vi "Delete_Crossconnection-1.vi"(5 "[IN] Row index\nInitial Point":i32, 7 "[IN] Column in\ndex Initial Point":i32, 9 "[IN] Indicies of Cross\nconnected Points":i32[](array[numeric]), 10 "[IN] The other point \nfor crossconnection found":bool, 11 "[IN] Track group":T1) -> (1 "[OUT] Track group":T1, 2 "[OUT] Column index\nCorrect initial point":i32, 3 "[OUT] Row index\nCorrect initial point":i32)   [LabVIEW 2013]
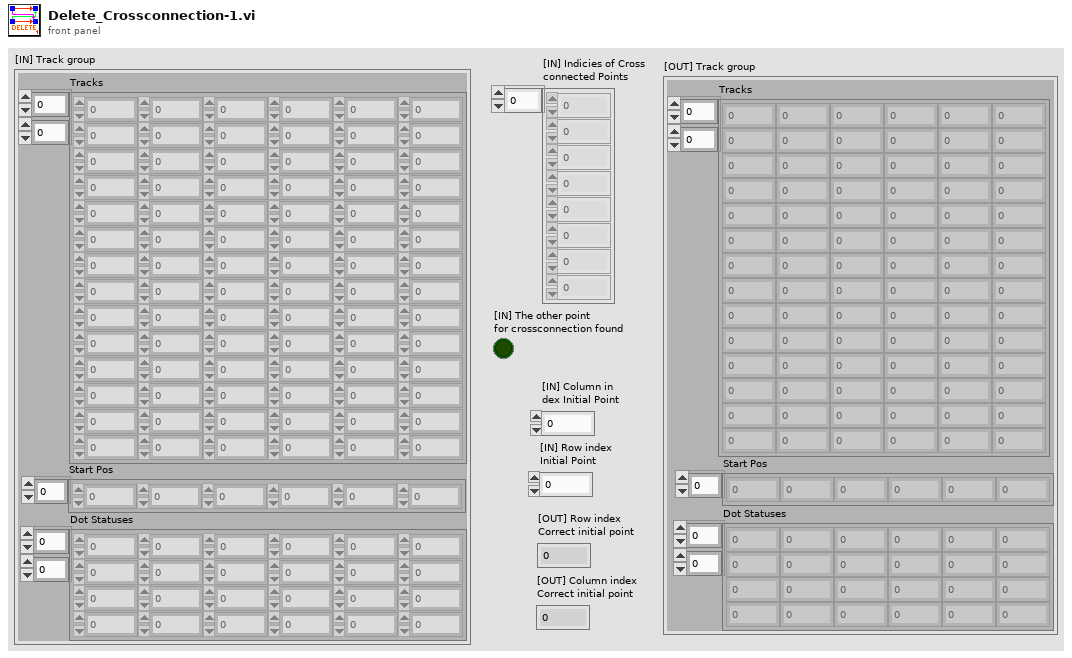
[diagram p1: front panel]
types:
  T1 = cluster{"Tracks":dbl[][], "Start Pos":i32[], "Dot Statuses":i16[][]}
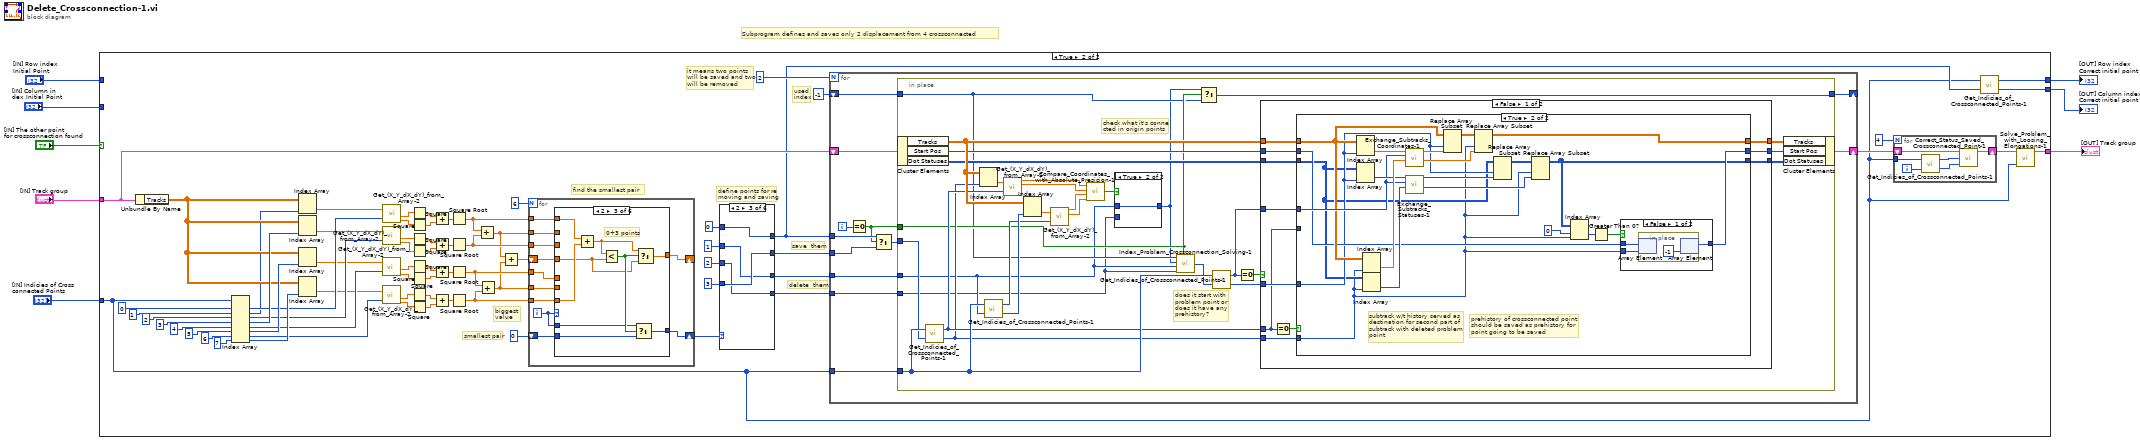
[diagram p0: block diagram]
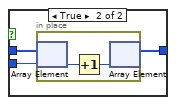
[diagram p4: hidden frame]
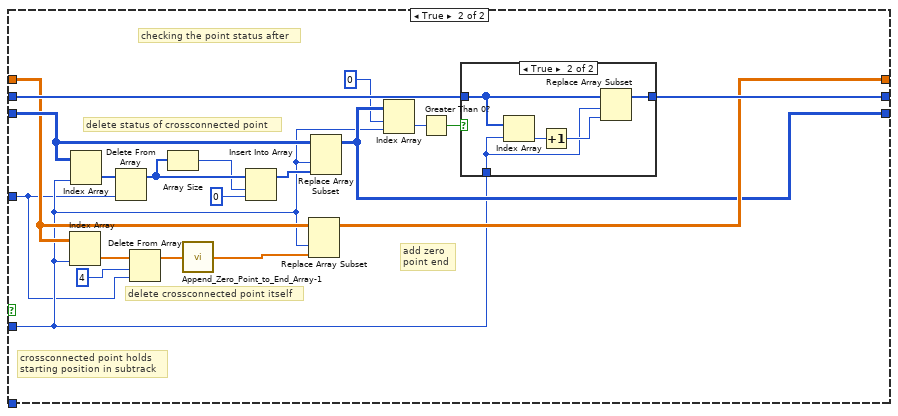
[diagram p5: hidden frame]
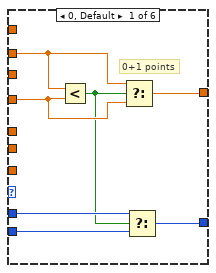
[diagram p13: hidden frame]
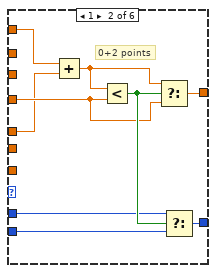
[diagram p14: hidden frame]
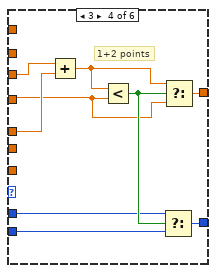
[diagram p15: hidden frame]
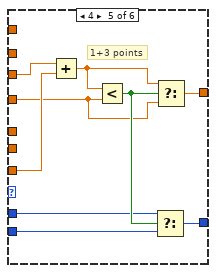
[diagram p16: hidden frame]
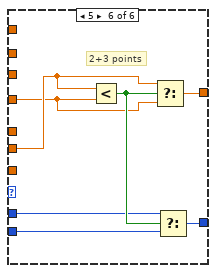
[diagram p17: hidden frame]
diagram:
  # "Subprogram defines and saves only 2 displacement from 4 crossconnected"
  n1 = case shown="True" "[IN] The other point \nfor crossconnection found" {
    tunnel: "[IN] Track group" -> [w11 w25]
    tunnel: "[IN] Indicies of Cross\nconnected Points" -> [_ w14]
    tunnel: [w11 w13] -> w5
    tunnel: [w10 w18] -> w4
    tunnel: [w9 w17] -> w3
    tunnel: "[IN] Row index\nInitial Point" -> [w10 _]
    tunnel: "[IN] Column in\ndex Initial Point" -> [w9 _]
    frame False {
    }
    frame True {
      # "used \nindex"
      # "it means two points\nwill be saved and two\nwill be removed"
      # "define points for re\nmoving and saving"
      # "delete  them"
      # "save  them"
      # "smallest pair"
      # "biggest \nvalue"
      # "find the smallest pair"
      n2 = Unbundle By Name(w25) -> ("Tracks"=w70:dbl[][])
      n3 = Index Array(array=w14, index #1=0 ("index"), index #2=1 ("index"), index #3=2 ("index"), index #4=3 ("index"), index #5=4 ("index"), index #6=5 ("index"), index #7=6 ("index"), index #8=7 ("index")) -> (element #1=w67:i32, element #2=w30:i32, element #3=w65:i32, element #4=w72:i32, element #5=w63:i32, element #6=w71:i32, element #7=w61:i32, element #8=w69:i32)
      n4 = Index Array(array=w70, index (col)=w69) -> (element=w62:dbl[])  [unwired: 1 in]
      n5 = Index Array(array=w70, index (col)=w30) -> (element=w68:dbl[])  [unwired: 1 in]
      n6 = Index Array(array=w70, index (col)=w72) -> (element=w66:dbl[])  [unwired: 1 in]
      n7 = Index Array(array=w70, index (col)=w71) -> (element=w64:dbl[])  [unwired: 1 in]
      n8 = call "Get_(X_Y_dX_dY)_from_Array-2.vi"("(X,Y,dX,dY)"=w66, "Index of Displacement"=w65) -> ("dX"=w52:dbl, "dY"=w51:dbl)  [unwired: 2 out]
      n9 = call "Get_(X_Y_dX_dY)_from_Array-2.vi"("(X,Y,dX,dY)"=w64, "Index of Displacement"=w63) -> ("dX"=w47:dbl, "dY"=w46:dbl)  [unwired: 2 out]
      n10 = call "Get_(X_Y_dX_dY)_from_Array-2.vi"("(X,Y,dX,dY)"=w62, "Index of Displacement"=w61) -> ("dX"=w42:dbl, "dY"=w41:dbl)  [unwired: 2 out]
      n11 = call "Get_(X_Y_dX_dY)_from_Array-2.vi"("(X,Y,dX,dY)"=w68, "Index of Displacement"=w67) -> ("dX"=w57:dbl, "dY"=w56:dbl)  [unwired: 2 out]
      n12 = Square(x=w57) -> (x^2=w60:dbl)
      n13 = Square(x=w56) -> (x^2=w59:dbl)
      n14 = Square(x=w52) -> (x^2=w55:dbl)
      n15 = Square(x=w51) -> (x^2=w54:dbl)
      n16 = Square(x=w47) -> (x^2=w50:dbl)
      n17 = Square(x=w46) -> (x^2=w49:dbl)
      n18 = Square(x=w42) -> (x^2=w45:dbl)
      n19 = Square(x=w41) -> (x^2=w44:dbl)
      n20 = Add(x=w60, y=w59) -> (x+y=w58:dbl)
      n21 = Add(x=w55, y=w54) -> (x+y=w53:dbl)
      n22 = Add(x=w50, y=w49) -> (x+y=w48:dbl)
      n23 = Add(x=w45, y=w44) -> (x+y=w43:dbl)
      n24 = Square Root(x=w58) -> (sqrt(x)=w39:dbl)
      n25 = Square Root(x=w53) -> (sqrt(x)=w38:dbl)
      n26 = Square Root(x=w48) -> (sqrt(x)=w37:dbl)
      n27 = Square Root(x=w43) -> (sqrt(x)=w36:dbl)
      n28 = Add(x=w39, y=w38) -> (x+y=w33:dbl)
      n29 = Add(x=w37, y=w36) -> (x+y=w32:dbl)
      n30 = Add(x=w33, y=w32) -> (x+y=w35:dbl)
      n31 = for {
        N: 6 -> [_]
        tunnel: w39 -> [w233]
        tunnel: w38 -> [w232]
        tunnel: w37 -> [w227]
        tunnel: w36 -> [w226]
        shift-right: [w230] -> _
        shift-left: w35 -> [w235]
        tunnel: w33 -> [w234]
        tunnel: w32 -> [w225]
        shift-right: [w228] -> w31
        shift-left: 0 -> [w229]
        i -> [w231]
        n32 = case shown="2" w231 {
          tunnel: w235 -> [w241 w246 w254 w263 w272 w281]
          tunnel: w234 -> [w242 _ _ _ _ _]
          tunnel: w233 -> [_ w251 w256 _ _ _]
          tunnel: w232 -> [_ _ _ w265 w274 _]
          tunnel: w231 -> [w239 w248 w258 w267 w271 w284]
          tunnel: [w240 w243 w253 w262 w276 w280] -> w230
          tunnel: w229 -> [w238 w247 w257 w266 w270 w283]
          tunnel: [w237 w249 w252 w261 w275 w279] -> w228
          tunnel: w227 -> [_ w244 _ w264 _ _]
          tunnel: w226 -> [_ _ w255 _ w273 _]
          tunnel: w225 -> [_ _ _ _ _ w282]
          frame 0, Default {
            # "0+1 points"
            n33 = Less?(x=w242, y=w241) -> (x < y?=w236:bool)
            n34 = Select(t=w242, s=w236, f=w241) -> (s? t:f=w240:dbl)
            n35 = Select(t=w239, s=w236, f=w238) -> (s? t:f=w237:i32)
          }
          frame 1 {
            # "0+2 points"
            n36 = Add(x=w251, y=w244) -> (x+y=w245:dbl)
            n37 = Less?(x=w245, y=w246) -> (x < y?=w250:bool)
            n38 = Select(t=w245, s=w250, f=w246) -> (s? t:f=w243:dbl)
            n39 = Select(t=w248, s=w250, f=w247) -> (s? t:f=w249:i32)
          }
          frame 2 {
            # "0+3 points"
            n40 = Add(x=w256, y=w255) -> (x+y=w259:dbl)
            n41 = Less?(x=w259, y=w254) -> (x < y?=w260:bool)
            n42 = Select(t=w258, s=w260, f=w257) -> (s? t:f=w252:i32)
            n43 = Select(t=w259, s=w260, f=w254) -> (s? t:f=w253:dbl)
          }
          frame 3 {
            # "1+2 points"
            n44 = Add(x=w265, y=w264) -> (x+y=w268:dbl)
            n45 = Less?(x=w268, y=w263) -> (x < y?=w269:bool)
            n46 = Select(t=w267, s=w269, f=w266) -> (s? t:f=w261:i32)
            n47 = Select(t=w268, s=w269, f=w263) -> (s? t:f=w262:dbl)
          }
          frame 4 {
            # "1+3 points"
            n48 = Add(x=w274, y=w273) -> (x+y=w277:dbl)
            n49 = Less?(x=w277, y=w272) -> (x < y?=w278:bool)
            n50 = Select(t=w271, s=w278, f=w270) -> (s? t:f=w275:i32)
            n51 = Select(t=w277, s=w278, f=w272) -> (s? t:f=w276:dbl)
          }
          frame 5 {
            # "2+3 points"
            n52 = Less?(x=w282, y=w281) -> (x < y?=w285:bool)
            n53 = Select(t=w282, s=w285, f=w281) -> (s? t:f=w280:dbl)
            n54 = Select(t=w284, s=w285, f=w283) -> (s? t:f=w279:i32)
          }
        }
      }
      n55 = case shown="2" w31 {
        tunnel: 0 -> [w204 w208 w212 w214 w218 w222]
        tunnel: 1 -> [w203 w206 w210 w216 w220 w221]
        tunnel: 2 -> [w202 w207 w209 w215 w217 w224]
        tunnel: 3 -> [w201 w205 w211 w213 w219 w223]
        tunnel: [w204 w208 w212 w216 w220 w224] -> w19
        tunnel: [w203 w207 w211 w215 w219 w223] -> w20
        tunnel: [w202 w206 w210 w214 w218 w222] -> w24
        tunnel: [w201 w205 w209 w213 w217 w221] -> w23
        frame 0, Default {
        }
        frame 1 {
        }
        frame 2 {
        }
        frame 3 {
        }
        frame 4 {
        }
        frame 5 {
        }
      }
      n56 = for {
        N: 2 -> [_]
        tunnel: w14 -> [w97]
        tunnel: w19 -> [w92]
        tunnel: w20 -> [w91]
        tunnel: w24 -> [w96]
        tunnel: w23 -> [w95]
        shift-right: [w94] -> w22
        shift-left: w25 -> [w98]
        shift-right: [w88] -> _
        shift-left: -1 -> [w89]
        i -> [w93]
        n57 = Equal To 0?(x=w93) -> (x = 0?=w87:bool)
        n58 = Select(t=w92, s=w87, f=w91) -> (s? t:f=w90:i32)
        n59 = in-place {
          in-place-border: w97 -> [w118]
          in-place-border: w96 -> [w100]
          in-place-border: w95 -> [w99]
          in-place-border: w90 -> [w108]
          in-place-border: w89 -> [w103]
          in-place-border: [w105] -> w88
          in-place-border: w87 -> [w104]
          # "does it start with \nproblem point or\ndoes it have any \nprehistory?"
          # "check what it's conne\ncted in origin points"
          n60 = in-place-cluster #1(w98) -> ("Tracks"=w116:dbl[][], "Start Pos"=w115:i32[], "Dot Statuses"=w114:i16[][])
          n61 = call "Get_Indicies_of_Crossconnected_Points-1.vi"("[IN] Index of point"=w108, "[IN] Indicies of Cross\nconnected Points"=w118) -> ("[OUT] Column index"=w106:i32, "[OUT] Row index"=w107:i32)
          n62 = Index Array(array=w116, index (col)=w106) -> (element=w127:dbl[])  [unwired: 1 in]
          n63 = call "Get_Indicies_of_Crossconnected_Points-1.vi"("[IN] Index of point"=w100, "[IN] Indicies of Cross\nconnected Points"=w118) -> ("[OUT] Column index"=w126:i32, "[OUT] Row index"=w124:i32)
          n64 = call "Get_(X_Y_dX_dY)_from_Array-2.vi"("(X,Y,dX,dY)"=w127, "Index of Displacement"=w107) -> ("X"=w123:dbl, "Y"=w122:dbl)  [unwired: 2 out]
          n65 = Index Array(array=w116, index (col)=w126) -> (element=w125:dbl[])  [unwired: 1 in]
          n66 = call "Get_(X_Y_dX_dY)_from_Array-2.vi"("(X,Y,dX,dY)"=w125, "Index of Displacement"=w124) -> ("X"=w121:dbl, "Y"=w120:dbl)  [unwired: 2 out]
          n67 = call "Compare_Coordinates_with_Absolute_Presicion-1.vi"("X 1"=w123, "Y 1"=w122, "X 2"=w121, "Y 2"=w120) -> ("[OUT] Same coordinates?"=w119:bool)  [unwired: 1 in]
          n68 = case shown="True" w119 {
            tunnel: w100 -> [_ w200]
            tunnel: w99 -> [w199 _]
            tunnel: [w199 w200] -> w102
            frame False {
            }
            frame True {
            }
          }
          n69 = call "Index_Problem_Crossconnection_Solving-1.vi"("[IN] Used Index"=w103, "[IN] Defined Index"=w102, "[IN] 1st Index for Deletion"=w100, "[IN] 2nd Index for Deletion"=w99, "[IN] Is it first step?"=w104) -> ("[OUT] Index of Track wi\nth Point For Deletion"=w101:i32)
          n70 = Select(t=w102, s=w104, f=w103) -> (s? t:f=w105:i32)
          n71 = call "Get_Indicies_of_Crossconnected_Points-1.vi"("[IN] Index of point"=w101, "[IN] Indicies of Cross\nconnected Points"=w118) -> ("[OUT] Column index"=w113:i32, "[OUT] Row index"=w111:i32)
          n72 = Equal To 0?(x=w111) -> (x = 0?=w117:bool)
          n73 = case shown="False" w117 {
            tunnel: w116 -> [w137 w182]
            tunnel: w115 -> [w136 w192]
            tunnel: w114 -> [w135 w187]
            tunnel: w113 -> [w130 w177]
            tunnel: [w133 w191] -> w112
            tunnel: w111 -> [w129 w174]
            tunnel: [w134 w180] -> w110
            tunnel: [w132 w178] -> w109
            tunnel: w107 -> [w128 _]
            tunnel: w106 -> [w131 _]
            frame False {
              n74 = Equal To 0?(x=w128) -> (x = 0?=w138:bool)
              n75 = case shown="True" w138 {
                tunnel: w137 -> [w141 w158]
                tunnel: w136 -> [w140 w149]
                tunnel: w135 -> [w139 w146]
                tunnel: [w141 w154] -> w134
                tunnel: [w140 w147] -> w133
                tunnel: [w139 w145] -> w132
                tunnel: w131 -> [_ w144]
                tunnel: w130 -> [_ w148]
                tunnel: w129 -> [_ w159]
                tunnel: w128 -> [_ _]
                frame False {
                  # "I suppose that tracking algorithm will be able to resolve such problem in this case"
                }
                frame True {
                  # "subtrack w/t history served as \ndestination for second part of \nsubtrack with deleted problem \npoint"
                  # "prehistory of crossconnected point \nshould be saved as prehistory for \npoint going to be saved"
                  n76 = Index Array(array=w158, index (col)=w148) -> (element=w163:dbl[])  [unwired: 1 in]
                  n77 = Index Array(array=w146, index (col)=w148) -> (element=w161:i16[])  [unwired: 1 in]
                  n78 = Index Array(array=w158, index (col)=w144) -> (element=w162:dbl[])  [unwired: 1 in]
                  n79 = Index Array(array=w146, index (col)=w144) -> (element=w160:i16[])  [unwired: 1 in]
                  n80 = call "Exchange_Subtracks_Coordinates-1.vi"("[IN] Subtrack wit\nhout prehistory"=w162, "[IN] Row index \nProblem Point"=w159, "[IN] Subtrack \nwith problem"=w163) -> ("[OUT] Reconnected subtrack\n(posthistory after deleted \ncrossconnected point)"=w155:dbl[], "[OUT] Reconnected subtrack\nPrehistory + alternative prob\nlem point"=w157:dbl[])  [unwired: 3 in]
                  n81 = call "Exchange_Subtracks_Statuses-1.vi"("[IN] Statuses wit\nhout prehistory"=w160, "[IN] Row index \nProblem Point"=w159, "[IN] Statuses\nwith problem"=w161) -> ("[OUT] Reconnected statuses\n(posthistory after deleted \ncrossconnected point)"=w151:i16[], "[OUT] Reconnected statuses\nPrehistory + alternative prob\nlem point"=w153:i16[])  [unwired: 3 in]
                  n82 = Replace Array Subset(array=w158, new element=w157, index (col)=w148) -> (w156:dbl[][])  [unwired: 1 in]
                  n83 = Replace Array Subset(array=w156, new element=w155, index (col)=w144) -> (w154:dbl[][])  [unwired: 1 in]
                  n84 = Replace Array Subset(array=w146, new element=w153, index (col)=w148) -> (w152:i16[][])  [unwired: 1 in]
                  n85 = Replace Array Subset(array=w152, new element=w151, index (col)=w144) -> (w145:i16[][])  [unwired: 1 in]
                  n86 = Index Array(array=w145, index (row)=0 ("disabled index (row)"), index (col)=w144) -> (element=w150:i16)
                  n87 = Greater Than 0?(x=w150) -> (x > 0?=w142:bool)
                  n88 = case shown="False" w142 {
                    tunnel: w149 -> [w166 w170]
                    tunnel: w144 -> [w165 w169]
                    tunnel: [w164 w168] -> w147
                    frame False {
                      n89 = in-place {
                        n90 = in-place-array #2(w166, w165) -> ()  [unwired: 1 out]
                        n91 = in-place-array #2(-1) -> (w164:i32[])  [unwired: 1 out]
                      }
                    }
                    frame True {
                      n92 = in-place {
                        n93 = in-place-array #3(w170, w169) -> (w172:i32)
                        n94 = Increment(x=w172) -> (x+1=w171:i32)
                        n95 = in-place-array #3(w171) -> (w168:i32[])  [unwired: 1 out]
                      }
                    }
                  }
                }
              }
            }
            frame True {
              # "add zero \npoint end"
              # "checking the point status after"
              # "delete crossconnected point itself"
              # "delete status of crossconnected point"
              # "crossconnected point holds \nstarting position in subtrack"
              n96 = Index Array(array=w182, index (col)=w177) -> (element=w185:dbl[])  [unwired: 1 in]
              n97 = Index Array(array=w187, index (col)=w177) -> (element=w190:i16[])  [unwired: 1 in]
              n98 = Delete From Array(array=w190, index=w174) -> (array with subset deleted=w189:i16[])  [unwired: 1 in, 1 out]
              n99 = Delete From Array(array=w185, length=4, index=w174) -> (array with subset deleted=w183:dbl[])  [unwired: 1 out]
              n100 = Array Size(array=w189) -> (size(s)=w179:i32)
              n101 = call "Append_Zero_Point_to_End_Array-1.vi"("[IN] Array with \nDisplacements"=w183) -> ("[OUT] Array with \nAppended Point"=w181:dbl[])
              n102 = Insert Into Array(array=w189, index=w179, new element=i16 0 ("new element/subarray")) -> (w186:i16[])
              n103 = Replace Array Subset(array=w182, new element=w181, index (col)=w177) -> (w180:dbl[][])  [unwired: 1 in]
              n104 = Replace Array Subset(array=w187, new element=w186, index (col)=w177) -> (w178:i16[][])  [unwired: 1 in]
              n105 = Index Array(array=w178, index (row)=0 ("disabled index (row)"), index (col)=w177) -> (element=w176:i16)
              n106 = Greater Than 0?(x=w176) -> (x > 0?=w175:bool)
              n107 = case shown="True" w175 {
                tunnel: w192 -> [w193 w198]
                tunnel: [w193 w195] -> w191
                tunnel: w177 -> [_ w194]
                frame False {
                }
                frame True {
                  n108 = Index Array(array=w198, index=w194) -> (element=w197:i32)
                  n109 = Increment(x=w197) -> (x+1=w196:i32)
                  n110 = Replace Array Subset(array=w198, new element=w196, index=w194) -> (w195:i32[])
                }
              }
            }
          }
          n111 = in-place-cluster #1("Tracks"=w110, "Start Pos"=w112, "Dot Statuses"=w109) -> (w94:T1)
        }
      }
      n112 = for {
        N: 4 -> [_]
        shift-right: [w85] -> w15
        shift-left: w22 -> [w86]
        tunnel: w14 -> [w82]
        i -> [w81]
        n113 = call "Get_Indicies_of_Crossconnected_Points-1.vi"("[IN] Index of point"=w81, "[IN] Indicies of Cross\nconnected Points"=w82) -> ("[OUT] Column index"=w83:i32, "[OUT] Row index"=w84:i32)
        n114 = call "Correct_Status_Saved_Crossconnected_Point-1.vi"("[IN] Column index"=w83, "[IN] Row index"=w84, "[IN] Track group"=w86) -> ("[OUT] Track group"=w85:T1)  [unwired: 2 in]
      }
      n115 = call "Get_Indicies_of_Crossconnected_Points-1.vi"("[IN] Index of point"=w19, "[IN] Indicies of Cross\nconnected Points"=w14) -> ("[OUT] Column index"=w17:i32, "[OUT] Row index"=w18:i32)
      n116 = call "Solve_Problem_with_Loosing_Elongations-1.vi"("[IN] Indicies of Cross\nconnected Points"=w14, "[IN] Track group"=w15) -> ("[OUT] Track group"=w13:T1)  [unwired: 3 in]
    }
  }
  "[OUT] Track group" <- w5
  "[OUT] Row index\nCorrect initial point" <- w4
  "[OUT] Column index\nCorrect initial point" <- w3
